vi "BotSpeak_HTTP.vi"(0 "BotSpeak File Name":path, 1 "URL":string, 2 "BotSpeak Code":string, 3 "cookie file":path) -> (7 "connection\nerror":errorcluster, 8 "file error":errorcluster)   [LabVIEW 2014]
uses:
  <vilib>/httpClient/POSTFile.vi
  <vilib>/httpClient/LabVIEWHTTPClient.lvlib
panel:
  out "result string":string
  out "headers":string
  out "body":string
  # "SET DIO[1],1"
  # "192.168.2.3:2012"
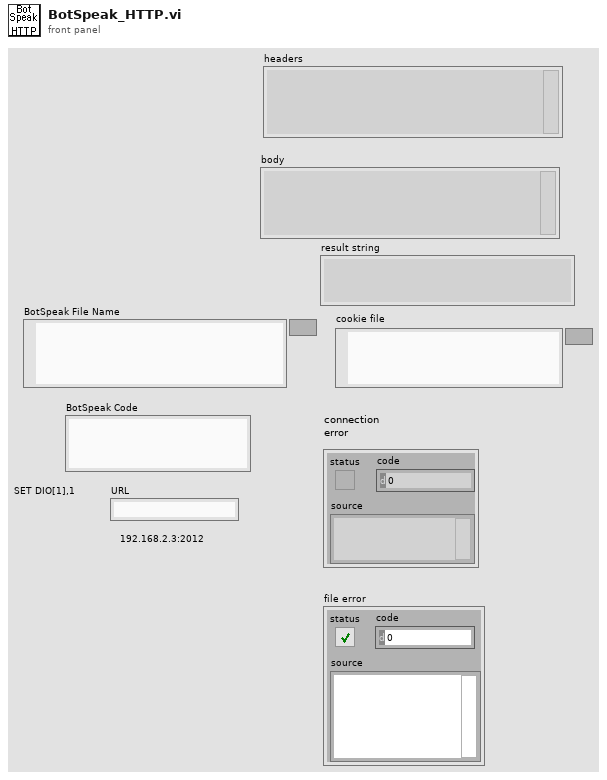
[diagram p1: front panel]
types:
  T1 = typedef "LabVIEWHTTPClient.lvlib/ClientHandle.ctl" = refnum<k1>
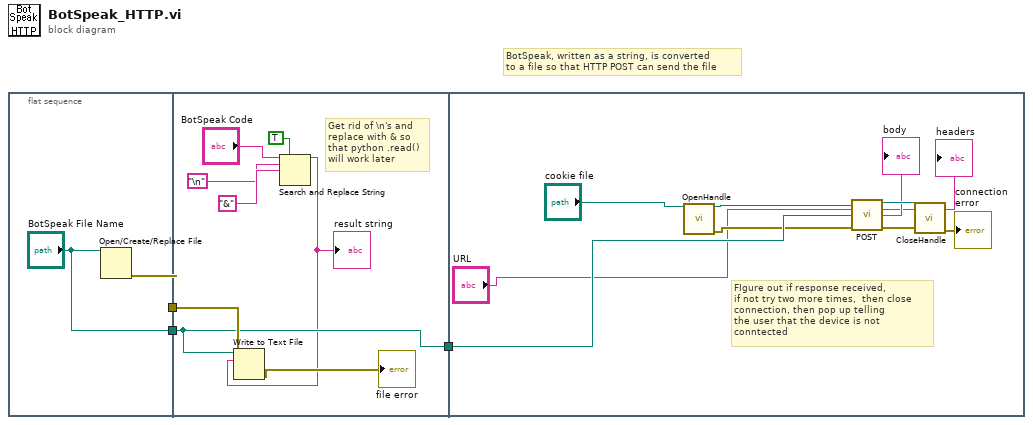
[diagram p0: block diagram]
diagram:
  # "BotSpeak, written as a string, is converted\nto a file so that HTTP POST can send the file"
  n1 = flat-sequence {
    tunnel: ["BotSpeak File Name"] -> w2
    tunnel: [w5] -> w1
    tunnel: [w11] -> w3
    tunnel: w2 -> [w11]
    tunnel: w1 -> [w13]
    tunnel: w3 -> [w21]
    frame #0 {
      n2 = Open/Create/Replace File(file path (use dialog)="BotSpeak File Name") -> (error out=w5:errorcluster)  [unwired: 5 in, 2 out]
    }
    frame #1 {
      # "Get rid of \\n's and\nreplace with & so \nthat python .read()\nwill work later"
      n3 = Search and Replace String(replace all?=TRUE ("replace all? (F)"), input string="BotSpeak Code", search string="\n", replace string="&" ("replace string (\"\")")) -> (result string=w7:string)  [unwired: 4 in, 3 out]
      "result string" <- w7
      n4 = Write to Text File(file (use dialog)=w11, text=w7, error in=w13) -> (error out=→"file error":errorcluster)  [unwired: 1 in, 2 out]
    }
    frame #2 {
      # "FIgure out if response received, \nif not try two more times,  then close \nconnection, then pop up telling\nthe user that the device is not \nconntected"
      n5 = call <vilib>:"OpenHandle.vi"("cookie file"="cookie file") -> ("client handle out"=w20:T1, "error out"=w19:errorcluster)  [unwired: 13 in]
      n6 = call-poly <vilib>:"POST.vi"("client handle"=w20, "url"="URL", "file"=w21, "error in (no error)"=w19) -> ("client handle out"=w18:T1, "headers"=→"headers":string, "body"=→"body":string, "error out"=w22:errorcluster)  [unwired: 8 in]
      n7 = call <vilib>:"CloseHandle.vi"("client handle"=w18, "error in (no error)"=w22) -> ("error out"=→"connection\nerror":errorcluster)  [unwired: 13 in]
    }
  }
